vi "CalcSampleVDC.vi"(8 "Rp":dbl format="%#_13g", 9 "Rl":dbl format="%#_13g", 10 "VDC (V)":dbl format="%#_13g", 11 "Sample Resistance (Ohms)":dbl format="%#_13g") -> (3 "Sample VDC (V)":dbl)   [LabVIEW 2016]
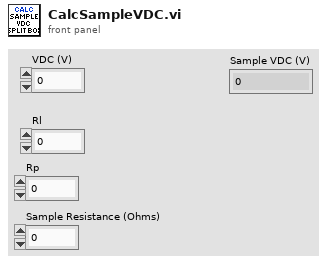
[diagram p1: front panel]
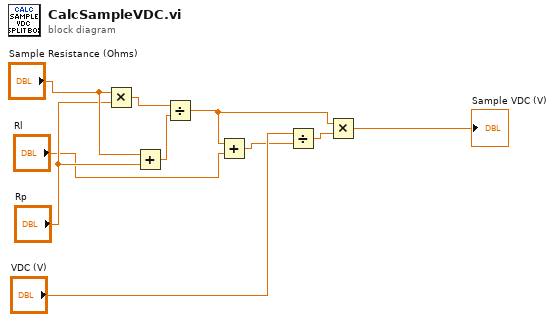
[diagram p0: block diagram]
diagram:
  n1 = Multiply(x="Sample Resistance (Ohms)", y="Rp") -> (x*y=w10:dbl)
  n2 = Add(x="Sample Resistance (Ohms)", y="Rp") -> (x+y=w7:dbl)
  n3 = Divide(x=w10, y=w7) -> (x/y=w2:dbl)
  n4 = Add(x=w2, y="Rl") -> (x+y=w4:dbl)
  n5 = Divide(x="VDC (V)", y=w4) -> (x/y=w3:dbl)
  n6 = Multiply(x=w2, y=w3) -> (x*y=→"Sample VDC (V)":dbl)
